vi "saveDataNodeEnd.vi"(8 "error in (no error)":errorcluster, 9 "indent":i32, 10 "XML Refnum in":refnum<file>, 11 "PWM in":refnum<class "PWM.lvclass">) -> (0 "error out":errorcluster, 2 "XML Refnum out":refnum<file>, 3 "PWM out":refnum<class "PWM.lvclass">)   [LabVIEW 2013, in "PWM.lvclass"]
doc: "Ends the process of saving a xceData Node to an XML formatted file."
uses:
  PWM.lvclass
  Channel/Channel.lvclass
  xCE/xceNode/xceNode.lvclass
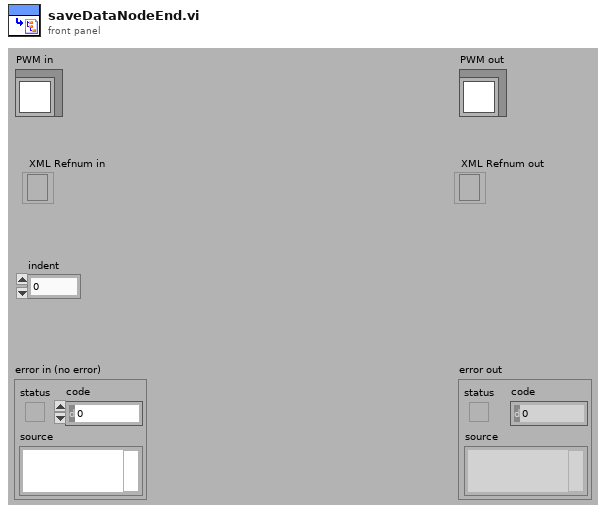
[diagram p1: front panel]
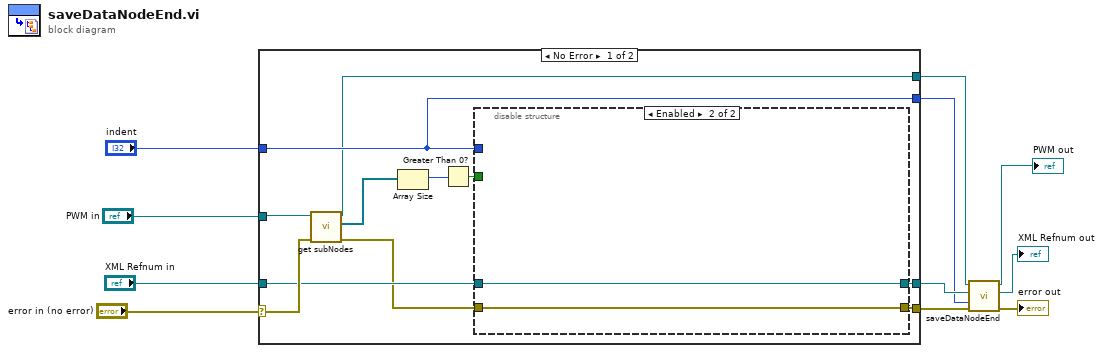
[diagram p0: block diagram]
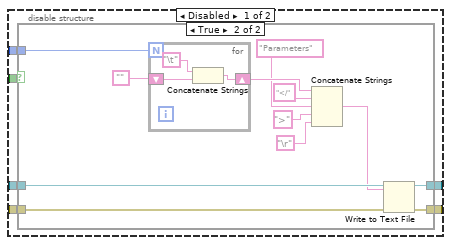
[diagram p2: hidden frame]
diagram:
  n1 = case shown="No Error" "error in (no error)" {
    selector: "error in (no error)" -> [w22 w48]
    tunnel: "PWM in" -> [w21 w51]
    tunnel: "indent" -> [w13 w50]
    tunnel: "XML Refnum in" -> [w17 w49]
    tunnel: [w14 w49] -> w5
    tunnel: [w13 w50] -> w4
    tunnel: [w12 w51] -> w2
    tunnel: [w15 w48] -> w1
    frame No Error {
      n2 = call "get subNodes.vi"("error in (no error)"=w22, "xceNode in"=w21) -> ("error out"=w16:errorcluster, "subNodes[]*"=w20:refnum<data-value>[], "xceNode out"=w12:refnum<class "PWM.lvclass">)  [unwired: 7 in]
      n3 = Array Size(array=w20) -> (size(s)=w19:i32)
      n4 = Greater Than 0?(x=w19) -> (x > 0?=w18:bool)
      n5 = disable-structure shown="Enabled" {
        disable-tunnel: w18 -> [w28 _]
        disable-tunnel: w17 -> [w27 w47]
        disable-tunnel: w16 -> [w26 w46]
        disable-tunnel: [w25 w46] -> w15
        disable-tunnel: [w24 w47] -> w14
        disable-tunnel: w13 -> [w23 _]
        frame Disabled {
          n6 = case shown="True" w28 {
            tunnel: w23 -> [_ w37]
            tunnel: w27 -> [w30 w35]
            tunnel: w26 -> [w29 w33]
            tunnel: [w29 w32] -> w25
            tunnel: [w30 w31] -> w24
            frame False {
            }
            frame True {
              n7 = for {
                N: w37 -> [_]
                shift-right: [w45] -> w38
                shift-left: "" -> [w44]
                n8 = Concatenate Strings("\t", w44) -> (w45:string)
              }
              n9 = Concatenate Strings(w38, "</", "Parameters" ("string"), ">", "\r") -> (w34:string)
              n10 = Write to Text File(file (use dialog)=w35, text=w34, error in=w33) -> (refnum out=w31:refnum<file>, error out=w32:errorcluster)  [unwired: 1 in, 1 out]
            }
          }
        }
        frame Enabled {
        }
      }
    }
    frame Error {
    }
  }
  n11 = call-parent "saveDataNodeEnd.vi"("error in (no error)"=w1, "indent"=w4, "XML Refnum in"=w5, "xceDataNode in"=w2) -> ("error out"=→"error out":errorcluster, "XML Refnum out"=→"XML Refnum out":refnum<file>, "xceDataNode out"=→"PWM out":refnum<class "PWM.lvclass">)  [unwired: 5 in]
